vi "STRUCT_2_STAGE.vi"(8 "Dataflow In":errorcluster) -> (0 "Dataflow Out":errorcluster)   [LabVIEW 2019]
panel:
  # "*******************************************************************\nBiogas Plant Control\n\nAuthor: Paul Zügel\nGCSC-Frankfurt am Main 2020\n\n*******************************************************************"
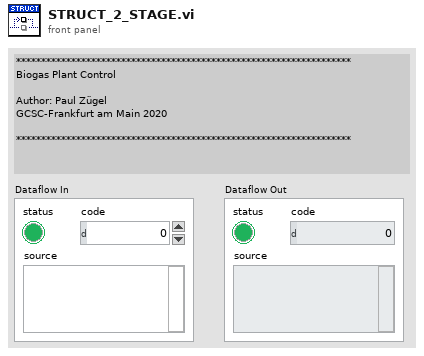
[diagram p1: front panel]
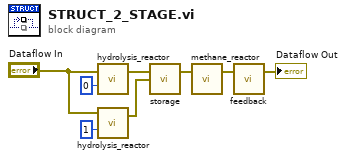
[diagram p0: block diagram]
diagram:
  n1 = call "hydrolysis_reactor.vi"("#"=i16 0, "Dataflow In"="Dataflow In") -> ("Dataflow Out"=w7:errorcluster)  [unwired: 2 in]
  n2 = call "hydrolysis_reactor.vi"("#"=i16 1, "Dataflow In"="Dataflow In") -> ("Dataflow Out"=w6:errorcluster)  [unwired: 2 in]
  n3 = call "storage.vi"("Dataflow In #3"=w6, "Dataflow In #1"=w7) -> ("Dataflow Out"=w5:errorcluster)  [unwired: 2 in]
  n4 = call "methane_reactor.vi"("Dataflow In"=w5) -> ("Dataflow Out"=w2:errorcluster)  [unwired: 2 in]
  n5 = call "feedback.vi"("Dataflow In"=w2) -> ("Dataflow Out"=→"Dataflow Out":errorcluster)  [unwired: 2 in]
